vi "Sandbox.vi"() -> ()   [LabVIEW 2019, in "OscillationDetector.lvclass"]
uses:
  OscillationDetector.lvclass
  DATA Oscill.ctl
  OscillationDetector.lvclass/OscillationDetector.ctl
panel:
  in  "milliseconds to wait":u32=10
  in  "N":i32=5000
  out "Waveform Chart":dbl(graph)
  out "LOWER TH":dbl
  out "UPPER TH":dbl
  out "DATA PERIOD":T1
  out "DATA N":T1
  in  "Offset":dbl
  in  "A":dbl
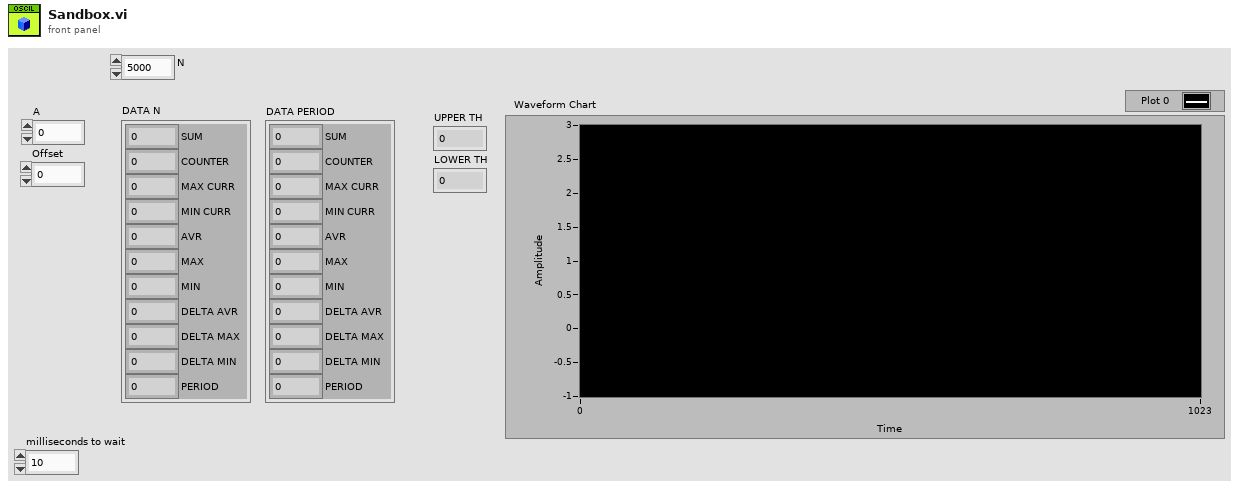
[diagram p1: front panel]
types:
  T1 = typedef "DATA Oscill.ctl" = cluster{"SUM":dbl, "COUNTER":dbl, "MAX CURR":dbl, "MIN CURR":dbl, "AVR":dbl, "MAX":dbl, "MIN":dbl, "DELTA AVR":dbl, "DELTA MAX":dbl, "DELTA MIN":dbl, "PERIOD":dbl}
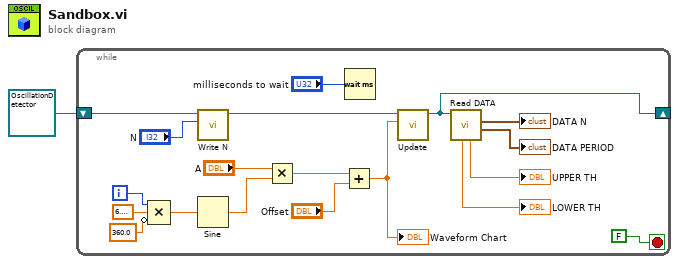
[diagram p0: block diagram]
diagram:
  n1 = while {
    shift-right: [w9] -> _
    shift-left: refnum<class "OscillationDetector.lvclass"> refnum ("OscillationDetector in") -> [w12]
    i -> [w20]
    stop <- FALSE stop-if-true
    n2 = Compound Arithmetic op=MULTIPLY(w20, 6.283185307179586, invert 360.0 ("value")) -> (w18:dbl)
    n3 = call "Write N.vi"("N"="N", "OscillationDetector in"=w12) -> ("OscillationDetector out"=w11:refnum<class "OscillationDetector.lvclass">)  [unwired: 9 in]
    n4 = Sine(x=w18) -> (sin(x)=w17:dbl)
    n5 = Multiply(x="A", y=w17) -> (x*y=w15:dbl)
    n6 = Add(x=w15, y="Offset") -> (x+y=w4:dbl)
    "Waveform Chart" <- w4
    n7 = Wait (ms)(milliseconds to wait="milliseconds to wait") -> ()  [unwired: 1 out]
    n8 = call "Update.vi"("Value"=w4, "OscillationDetector in"=w11) -> ("OscillationDetector out"=w9:refnum<class "OscillationDetector.lvclass">)  [unwired: 9 in]
    n9 = call "Read DATA.vi"("OscillationDetector in"=w9) -> ("DATA PERIOD"=→"DATA PERIOD":T1, "DATA N"=→"DATA N":T1, "UPPER TH"=→"UPPER TH":dbl, "LOWER TH"=→"LOWER TH":dbl)  [unwired: 7 in]
  }
